vi "Add Resource (IQ Impairments).vi"(0 "instance":u8, 1 "channel":u8, 2 "gen in":refnum<class "niUSRP Tx DSP v2 FPGA.lvclass">, 3 "collection builder in":refnum<class "Collection Builder.lvclass">, 5 "IP enabled":bool) -> (13 "gen out":refnum<class "niUSRP Tx DSP v2 FPGA.lvclass">, 14 "collection builder out":refnum<class "Collection Builder.lvclass">)   [LabVIEW 2025, in "niUSRP Tx DSP v2 FPGA.lvclass"]
uses:
  niUSRP Tx DSP v2 FPGA.lvclass
  <instrlib>/_niInstr/Instruction Framework/v1/FPGA/Collection Builder/Collection Builder.lvclass
  <instrlib>/_niInstr/DSP Control/Interface/v1/FPGA/IQ Impairments/IQ 18-bit/IQ Impairments Interface (18-bit).lvclass
  <instrlib>/_niInstr/DSP Control/Common/v2/FPGA/IQ Impairments/IQ 18-bit/IQ Impairments (18-bit).lvclass
  C:/Program Files/NI/LVAddons/niidl/1/instr.lib/_niInstr/DSP Control/Interface/v1/FPGA/IQ Impairments/IQ 18-bit/IQ Impairments Interface (18-bit).lvclass
  <instrlib>/_niInstr/Instruction Framework/v1/FPGA/Helper Classes/Single Address Space Collection/Single Address Space Collection.lvclass
  C:/Program Files/NI/LVAddons/niidl/1/instr.lib/_niInstr/Instruction Framework/v1/FPGA/Interfaces/Address Space Collection/Address Space Collection.lvclass
  <instrlib>/_niInstr/Basic Elements/v1/FPGA/niInstr Basic Elements v1 FPGA.lvlib
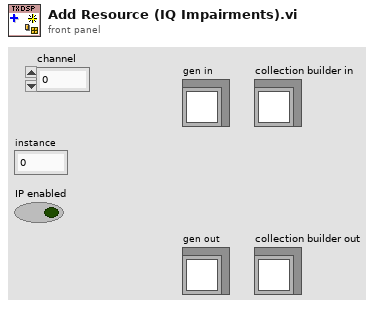
[diagram p1: front panel]
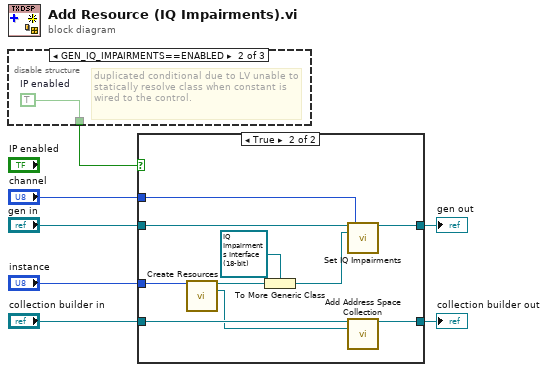
[diagram p0: block diagram]
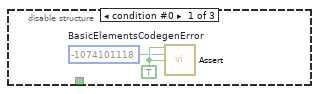
[diagram p2: hidden frame]
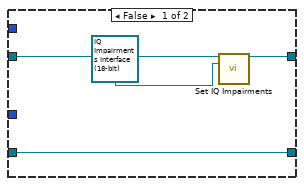
[diagram p4: hidden frame]
diagram:
  n1 = disable-structure shown="GEN_IQ_IMPAIRMENTS==ENABLED" {
    disable-tunnel: [_ w10 _] -> w2
    frame condition #0 {
      w9 = TRUE ("assert")
      w8 = -1074101118  # BasicElementsCodegenError
      n2 = call <instrlib>:"Assert.vi"("assert"=w9, "error code"=w8, "enable show error"=w9) -> ()  [unwired: 13 in]
    }
    frame condition #1 {
      w10 = TRUE  # IP enabled
      # "duplicated conditional due to LV unable to statically resolve class when constant is wired to the control."
    }
    frame condition #2 (active) {
    }
  }
  n3 = case shown="True" w2 {
    tunnel: "collection builder in" -> [w14 w24]
    tunnel: [w14 w23] -> w6
    tunnel: "instance" -> [_ w21]
    tunnel: "gen in" -> [w12 w17]
    tunnel: [w13 w18] -> w3
    tunnel: "channel" -> [_ w15]
    frame False {
      n4 = call-dynamic "Set IQ Impairments.vi"("gen in"=w12, "iq impairments"=refnum<class "IQ Impairments Interface (18-bit).lvclass"> refnum) -> ("gen out"=w13:refnum<class "niUSRP Tx DSP v2 FPGA.lvclass">)  [unwired: 13 in]
    }
    frame True {
      n5 = call <instrlib>:"Create Resources.vi"("instance"=w21) -> ("iq impairments"=w20:refnum<class "IQ Impairments (18-bit).lvclass">, "iq impairments registers"=w19:refnum<class "Single Address Space Collection.lvclass">)  [unwired: 13 in]
      n6 = To More Generic Class(target class=refnum<class "IQ Impairments Interface (18-bit).lvclass"> refnum ("iq impairments"), reference=w20) -> (generic class reference=w16:refnum<class "IQ Impairments Interface (18-bit).lvclass">)
      n7 = call-dynamic "Set IQ Impairments.vi"("gen in"=w17, "channel"=w15, "iq impairments"=w16) -> ("gen out"=w18:refnum<class "niUSRP Tx DSP v2 FPGA.lvclass">)  [unwired: 12 in]
      n8 = call <instrlib>:"Add Address Space Collection.vi"("collection builder in"=w24, "address space collection"=w19) -> ("collection builder out"=w23:refnum<class "Collection Builder.lvclass">)  [unwired: 13 in]
    }
  }
  "collection builder out" <- w6
  "gen out" <- w3
